vi "Execute Sequence Loop.vi"(4 "Sequence Progress":refnum<vi>, 8 "error in (no error)":errorcluster, 11 "class objects in":T1) -> (0 "error out":errorcluster, 3 "class objects Out":T1)   [LabVIEW 2011]
uses:
  Controls/Class Objects.ctl
  Modules/File/Configuration/Configuration.lvclass
  Modules/Hardware/Power Supply/Power Supply.lvclass
  Modules/Hardware/NMR/NMR.lvclass
  Modules/File/TDMS/TDMS.lvclass
  Controls/User Interface Action.ctl
  Controls/NMR Pulse Sequence Type.ctl
  Functional Globals/Pulse Parameters.ctl
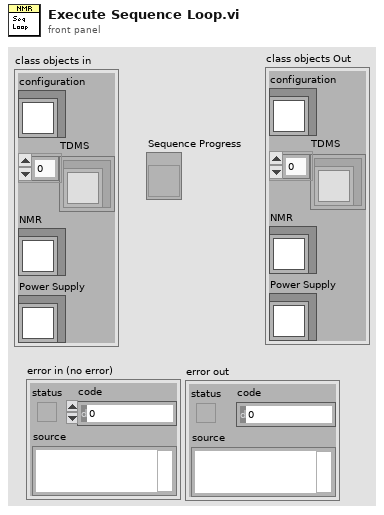
[diagram p1: front panel]
types:
  T1 = typedef "Class Objects.ctl" = cluster{"configuration":refnum<class "Configuration.lvclass">, "TDMS":refnum<class "TDMS.lvclass">[], "Power Supply":refnum<class "Power Supply.lvclass">, "NMR":refnum<class "NMR.lvclass">}
  T2 = typedef "NMR Pulse Sequence Type.ctl" = enum16{"90 Degree Sequence", "CPMG Pulse Sequence", "T1 Pulse Sequence"}
  T3 = typedef "Full_90 Degree Pulse Settings.ctl" = cluster{"Delay Settings":T4, "Preliminary Settings":T5, "Pulse Settings":T6, "Acquisition Settings":T7}
  T4 = typedef "90D_Delay Settings.ctl" = cluster{"Delay d1":dbl, "Delay d2":dbl, "d1 Unit":u8, "d2 Unit":u8}
  T5 = typedef "90D_Preliminary Settings.ctl" = cluster{"Nº of Scans (ns)":u16, "Pulse Frequency":dbl}
  T6 = typedef "90D_Pulse Settings.ctl" = cluster{"Duration Signal P1":dbl, "Power Level":u16, "Phase":u16, "P1 Units":u8}
  T7 = typedef "Acquisition Settings.ctl" = cluster{"Number Samples":u16, "Time Between Points":dbl, "Unit":u8}
  T8 = typedef "Full_CPMG Degree Pulse Settings.ctl" = cluster{"Acquisition Settings":T7, "Delay Settings":T9, "Preliminary Settings":T10, "Pulse Settings":T11}
  T9 = typedef "CPMG_Delay Settings.ctl" = cluster{"Delay d1":dbl, "Delay d2":dbl, "d1 Unit":u8, "d2 Unit":u8, "Delay d3":dbl, "d3 Unit":u8, "Delay d4":dbl, "d4 Unit":u8}
  T10 = typedef "CPMG_Preliminary Settings.ctl" = cluster{"Nº of Scans (ns)":u16, "Pulse Frequency":dbl, "Nº of Echoes (ne)":u16}
  T11 = typedef "CPMG_Pulse Settings.ctl" = cluster{"Duration Signal P1":dbl, "Power Level P1":u16, "Phase P1":u16, "P1 Unit":u8, "Duration Signal P2":dbl, "Power Level P2":u16, "Phase P2":u16, "P2 Unit":u8}
  T12 = typedef "Full_T1 Degree Pulse Settings.ctl" = cluster{"Preliminary Settings":T13, "Pulse Settings":T14, "Acquisition Settings":T7, "Delay Settings":T15}
  T13 = typedef "T1_Preliminary Settings.ctl" = cluster{"Nº of Scans (ns)":u16, "Pulse Frequency":dbl, "Nº of Vd":u16}
  T14 = typedef "T1_Pulse Settings.ctl" = cluster{"Duration Signal P2":dbl, "Power Level P2":u16, "Phase P2":u16, "P2 Unit":u8, "Duration Signal P1":dbl, "Power Level P1":u16, "Phase P1":u16, "P1 Unit":u8}
  T15 = typedef "T1_Delay Settings.ctl" = cluster{"Delay d1":dbl, "Delay d2":dbl, "d1 Unit":u8, "d2 Unit":u8, "Delay d30":dbl, "d30 Unit":u8, "Vd Unit":u8, "Vd Values":string}
  T16 = typedef "User Interface Action.ctl" = enum16{"Initialize", "Update Real Channel", "Update Imag Channel", "Update Re/Im channel @ Hardware Ctrl", "Pulse Sequence", "Visibility Front Panel Controls", "Report Custom Errors", "Set Pulse Sequence Type", "Update Pulse Timings", "Update Transfer Time", "Update Status Bar", "Set Sequence Progress", "Set 90 Degree Pulse Sequence Params", "Set CMPG Pulse Sequence Parms", "Set T1 Pulse Sequence Params", "Stop"}
  T17 = typedef "Pulse Parameters.ctl" = enum16{"Initialize", "Set T1 Pulse Settings", "Set 90 Degree Pulse Settings", "Set CPMG Pulse Settings", "Get T1 Settings", "Get CPMG Settings", "Get 90 Degree Settings"}
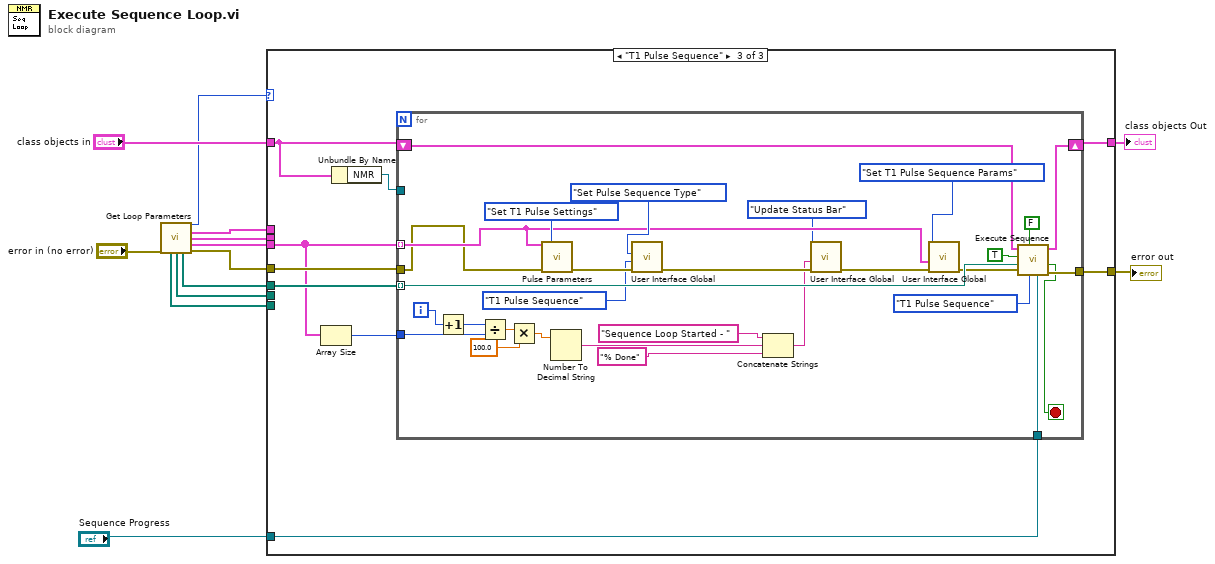
[diagram p0: block diagram]
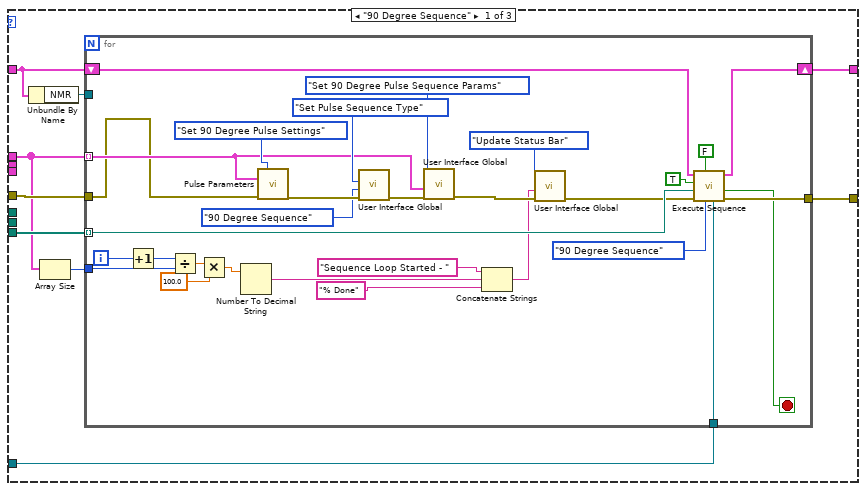
[diagram p2: hidden frame]
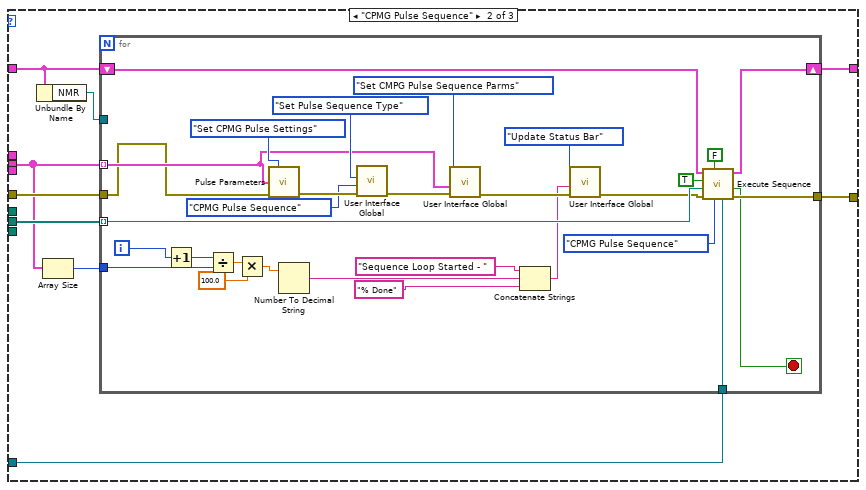
[diagram p3: hidden frame]
diagram:
  n1 = call "Get Loop Parameters.vi"("error in (no error)"="error in (no error)") -> ("Sequence Type"=w3:T2, "90Deg Pulse Sequence Array"=w7:T3[], "CPMG Pulse Sequence Array"=w9:T8[], "T1 Pulse Sequence Array"=w8:T12[], "90Deg path array"=w4:path[], "CPMG Path array"=w5:path[], "T1 path array"=w6:path[], "error out"=w11:errorcluster)  [unwired: 7 in]
  n2 = case shown="\"T1 Pulse Sequence\"" w3 {
    tunnel: w11 -> [w22 w61 w94]
    tunnel: "class objects in" -> [w17 w56 w96]
    tunnel: [w21 w60 w100] -> w10
    tunnel: w9 -> [_ w54 _]
    tunnel: w8 -> [_ _ w93]
    tunnel: w7 -> [w15 _ _]
    tunnel: w6 -> [_ _ w99]
    tunnel: w5 -> [_ w59 _]
    tunnel: w4 -> [w20 _ _]
    tunnel: "Sequence Progress" -> [w19 w58 w98]
    tunnel: [w18 w57 w97] -> w2
    frame "90 Degree Sequence" {
      n3 = Unbundle By Name(w17) -> ("NMR"=w16:refnum<class "NMR.lvclass">)
      n4 = Array Size(array=w15) -> (size(s)=w14:i32)
      n5 = for {
        tunnel: w22 -> [w24]
        shift-right: [w50] -> w18
        shift-left: w17 -> [w51]
        tunnel: [w48] -> w21
        tunnel: w15 -> [w38] mode=indexing
        tunnel: w20 -> [w46] mode=indexing
        tunnel: w19 -> [w44]
        tunnel: w16 -> [_]
        tunnel: w14 -> [w27]
        i -> [w26]
        stop <- w23 stop-if-true
        n6 = Increment(x=w26) -> (x+1=w25:i32)
        n7 = Divide(x=w25, y=w27) -> (x/y=w34:dbl)
        n8 = Multiply(x=w34, y=100.0) -> (x*y=w32:dbl)
        n9 = Number To Decimal String(number=w32) -> (decimal integer string=w29:string)  [unwired: 1 in]
        n10 = call "Pulse Parameters.vi"("action"=Pulse_Parameters."Set 90 Degree Pulse Settings", "90 Degree Pulse Sequence"=w38, "error in"=w24) -> ("error out"=w43:errorcluster)  [unwired: 5 in, 7 out]
        n11 = call "User Interface Global.vi"("error in"=w43, "data1"=NMR_Pulse_Sequence_Type."90 Degree Sequence" ("Pulse Sequence Type"), "action"=User_Interface_Action."Set Pulse Sequence Type") -> ("error out"=w42:errorcluster)  [unwired: 8 in]
        n12 = call "User Interface Global.vi"("error in"=w42, "data1"=w38, "action"=User_Interface_Action."Set 90 Degree Pulse Sequence Params") -> ("error out"=w36:errorcluster)  [unwired: 8 in]
        n13 = Concatenate Strings("Sequence Loop Started - ", w29, "% Done") -> (w28:string)
        n14 = call "User Interface Global.vi"("error in"=w36, "data1"=w28, "action"=User_Interface_Action."Update Status Bar") -> ("error out"=w35:errorcluster)  [unwired: 8 in]
        n15 = call "Execute Sequence.vi"("Sequence Progress"=w44, "Pulse Sequence Type"=NMR_Pulse_Sequence_Type."90 Degree Sequence", "Sum?"=FALSE, "error in (no error)"=w35, "file path (use dialog)"=w46, "Save File"=TRUE, "class objects in"=w51) -> ("error out"=w48:errorcluster, "Stop?"=w23:bool, "class objects out"=w50:T1)  [unwired: 1 in, 1 out]
      }
    }
    frame "CPMG Pulse Sequence" {
      n16 = Unbundle By Name(w56) -> ("NMR"=w55:refnum<class "NMR.lvclass">)
      n17 = Array Size(array=w54) -> (size(s)=w53:i32)
      n18 = for {
        tunnel: w61 -> [w76]
        shift-right: [w89] -> w57
        shift-left: w56 -> [w90]
        tunnel: [w87] -> w60
        tunnel: w54 -> [w78] mode=indexing
        tunnel: w59 -> [w86] mode=indexing
        tunnel: w58 -> [w83]
        tunnel: w55 -> [_]
        tunnel: w53 -> [w68]
        i -> [w67]
        stop <- w62 stop-if-true
        n19 = Increment(x=w67) -> (x+1=w69:i32)
        n20 = Divide(x=w69, y=w68) -> (x/y=w75:dbl)
        n21 = Multiply(x=w75, y=100.0) -> (x*y=w73:dbl)
        n22 = call "Pulse Parameters.vi"("action"=Pulse_Parameters."Set CPMG Pulse Settings", "CPMG Pulse Sequence"=w78, "error in"=w76) -> ("error out"=w82:errorcluster)  [unwired: 5 in, 7 out]
        n23 = Number To Decimal String(number=w73) -> (decimal integer string=w70:string)  [unwired: 1 in]
        n24 = call "User Interface Global.vi"("error in"=w82, "data1"=NMR_Pulse_Sequence_Type."CPMG Pulse Sequence" ("Pulse Sequence Type"), "action"=User_Interface_Action."Set Pulse Sequence Type") -> ("error out"=w81:errorcluster)  [unwired: 8 in]
        n25 = call "User Interface Global.vi"("error in"=w81, "data1"=w78, "action"=User_Interface_Action."Set CMPG Pulse Sequence Parms") -> ("error out"=w65:errorcluster)  [unwired: 8 in]
        n26 = Concatenate Strings("Sequence Loop Started - ", w70, "% Done") -> (w63:string)
        n27 = call "User Interface Global.vi"("error in"=w65, "data1"=w63, "action"=User_Interface_Action."Update Status Bar") -> ("error out"=w64:errorcluster)  [unwired: 8 in]
        n28 = call "Execute Sequence.vi"("Sequence Progress"=w83, "Pulse Sequence Type"=NMR_Pulse_Sequence_Type."CPMG Pulse Sequence", "Sum?"=FALSE, "error in (no error)"=w64, "file path (use dialog)"=w86, "Save File"=TRUE, "class objects in"=w90) -> ("error out"=w87:errorcluster, "Stop?"=w62:bool, "class objects out"=w89:T1)  [unwired: 1 in, 1 out]
      }
    }
    frame "T1 Pulse Sequence" {
      n29 = Array Size(array=w93) -> (size(s)=w92:i32)
      n30 = Unbundle By Name(w96) -> ("NMR"=w95:refnum<class "NMR.lvclass">)
      n31 = for {
        tunnel: w94 -> [w115]
        shift-right: [w128] -> w97
        shift-left: w96 -> [w129]
        tunnel: w93 -> [w117] mode=indexing
        tunnel: [w126] -> w100
        tunnel: w99 -> [w125] mode=indexing
        tunnel: w98 -> [w121]
        tunnel: w95 -> [_]
        tunnel: w92 -> [w103]
        i -> [w104]
        stop <- w101 stop-if-true
        n32 = Increment(x=w104) -> (x+1=w105:i32)
        n33 = Divide(x=w105, y=w103) -> (x/y=w111:dbl)
        n34 = Multiply(x=w111, y=100.0) -> (x*y=w109:dbl)
        n35 = call "Pulse Parameters.vi"("T1 Pulse Sequence"=w117, "action"=Pulse_Parameters."Set T1 Pulse Settings", "error in"=w115) -> ("error out"=w119:errorcluster)  [unwired: 5 in, 7 out]
        n36 = Number To Decimal String(number=w109) -> (decimal integer string=w106:string)  [unwired: 1 in]
        n37 = call "User Interface Global.vi"("error in"=w119, "data1"=NMR_Pulse_Sequence_Type."T1 Pulse Sequence" ("Pulse Sequence Type"), "action"=User_Interface_Action."Set Pulse Sequence Type") -> ("error out"=w113:errorcluster)  [unwired: 8 in]
        n38 = Concatenate Strings("Sequence Loop Started - ", w106, "% Done") -> (w102:string)
        n39 = call "User Interface Global.vi"("error in"=w113, "data1"=w102, "action"=User_Interface_Action."Update Status Bar") -> ("error out"=w112:errorcluster)  [unwired: 8 in]
        n40 = call "User Interface Global.vi"("error in"=w112, "data1"=w117, "action"=User_Interface_Action."Set T1 Pulse Sequence Params") -> ("error out"=w122:errorcluster)  [unwired: 8 in]
        n41 = call "Execute Sequence.vi"("Sequence Progress"=w121, "Pulse Sequence Type"=NMR_Pulse_Sequence_Type."T1 Pulse Sequence", "Sum?"=FALSE, "error in (no error)"=w122, "file path (use dialog)"=w125, "Save File"=TRUE, "class objects in"=w129) -> ("error out"=w126:errorcluster, "Stop?"=w101:bool, "class objects out"=w128:T1)  [unwired: 1 in, 1 out]
      }
    }
  }
  "error out" <- w10
  "class objects Out" <- w2
